vi "Send OOB TX.vi"(8 "error in (no error)":errorcluster, 11 "CIFCorePlugin in":refnum<class "CIFCorePlugin.lvclass">) -> (0 "error out":errorcluster, 3 "CIFCorePlugin out":refnum<class "CIFCorePlugin.lvclass">)   [LabVIEW 2021, in "CIFCorePlugin.lvclass"]
uses:
  CIFCorePlugin.lvclass
  CIFCorePlugin.lvclass/CIFCorePlugin.ctl
  CIFUtilities/CIFChannelMng/CIFChannelMng.lvclass/CIFChannelMng.ctl
  Common/Typedef/Plugin Overrides.ctl
  Common/Typedef/Timing Overrides.ctl
  Common/Typedef/Plugin Status.ctl
  Common/Typedef/Plugin State.ctl
  Common/Typedef/Timing Statistics.ctl
  Common/Typedef/Timing Stats Base.ctl
  Common/Typedef/FIFO Statistics.ctl
  Common/Typedef/Simple Error.ctl
  Common/Typedef/Monitor Doubles.ctl
  Common/Typedef/Monitor U64.ctl
  Common/Typedef/Monitor I64.ctl
  CIFUtilities/CIFOutOfBand/CIFOutOfBand.lvclass/CIFOutOfBand.ctl
  CIFUtilities/CIFOutOfBand/Write OOB DVR.vi
  CIFUtilities/CIFOutOfBand/Utilities/Command to Bitwise Command.vi
  CIFUtilities/CIFOutOfBand/Accessors/Read Local OOB Data.vi
  CIFUtilities/CIFOutOfBand/Accessors/Write Local OOB Data.vi
  CIFUtilities/CIFChannelMng/Accessors/Read Update OOB.vi
  CIFUtilities/CIFChannelMng/Accessors/Read Channel Status for OOB.vi
  CIFUtilities/CIFChannelMng/Accessors/Write Update OOB.vi
  OOB/OOB_Tx/CIFCoreOOB_Tx.lvclass
  D:/dev/CIF-LVCore/src/CIFUtilities/CIFOutOfBand/CIFOutOfBand.lvclass
  Common/CIFCoreCommon.lvlib
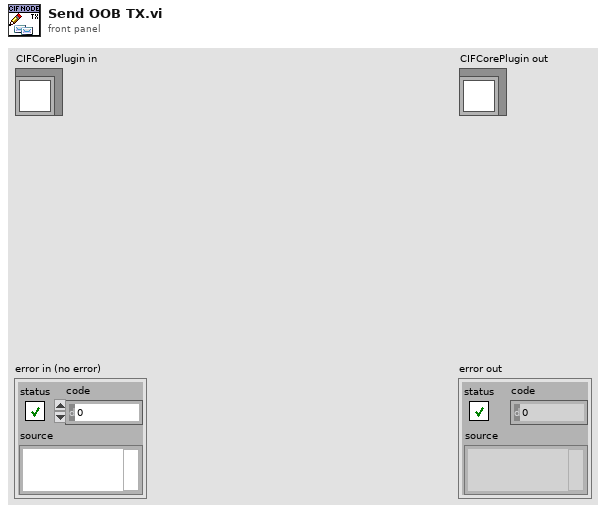
[diagram p1: front panel]
types:
  T1 = typedef "CIFCoreCommon.lvlib/Plugin Overrides.ctl" = cluster{"Timing Overrides":T2}
  T2 = typedef "CIFCoreCommon.lvlib/Timing Overrides.ctl" = cluster{"Override Timing":bool, "Skip Sleep":bool, "Period (s)":dbl}
  T3 = typedef "CIFCoreCommon.lvlib/Plugin Status.ctl" = cluster{"State":T4, "Timing Statistics (us)":T5, "FIFO Statistics (us)":T7, "error":T8, "Monitor Doubles":T9, "Monitor U64":T10, "Monitor I64":T11, "Cleanup":T6, "Create":i32, "Destroy":i32}
  T4 = typedef "CIFCoreCommon.lvlib/Plugin State.ctl" = enum32{"Null", "Creating", "Listening", "Running", "CleaningUp", "Destroying"}
  T5 = typedef "CIFCoreCommon.lvlib/Timing Statistics.ctl" = cluster{"Period":T6, "Wake Error":T6, "Execute":T6, "Housekeep":T6, "Idle":T6}
  T6 = typedef "CIFCoreCommon.lvlib/Timing Stats Base.ctl" = cluster{"Max":i32, "Min":i32}
  T7 = typedef "CIFCoreCommon.lvlib/FIFO Statistics.ctl" = cluster{"From T0":T6, "From Previous Plugin":T6, "Output Error":T6}
  T8 = typedef "CIFCoreCommon.lvlib/Simple Error.ctl" = cluster{"status":bool, "code":i32}
  T9 = typedef "CIFCoreCommon.lvlib/Monitor Doubles.ctl" = cluster{"1":dbl, "2":dbl, "3":dbl, "4":dbl}
  T10 = typedef "CIFCoreCommon.lvlib/Monitor U64.ctl" = cluster{"1":u64, "2":u64, "3":u64, "4":u64}
  T11 = typedef "CIFCoreCommon.lvlib/Monitor I64.ctl" = cluster{"1":i64, "2":i64, "3":i64, "4":i64}
  T12 = typedef "CIFChannelMng.lvclass/Channel List for OOB.ctl" = cluster{"Name":string, "Direction":T13, "Type":string, "Connected?":bool, "Connected Name":string, "Custom Config Data":u8[]}
  T13 = typedef "CIFChannels.lvclass/Direction.ctl" = enum16{"Publisher", "Subscriber"}
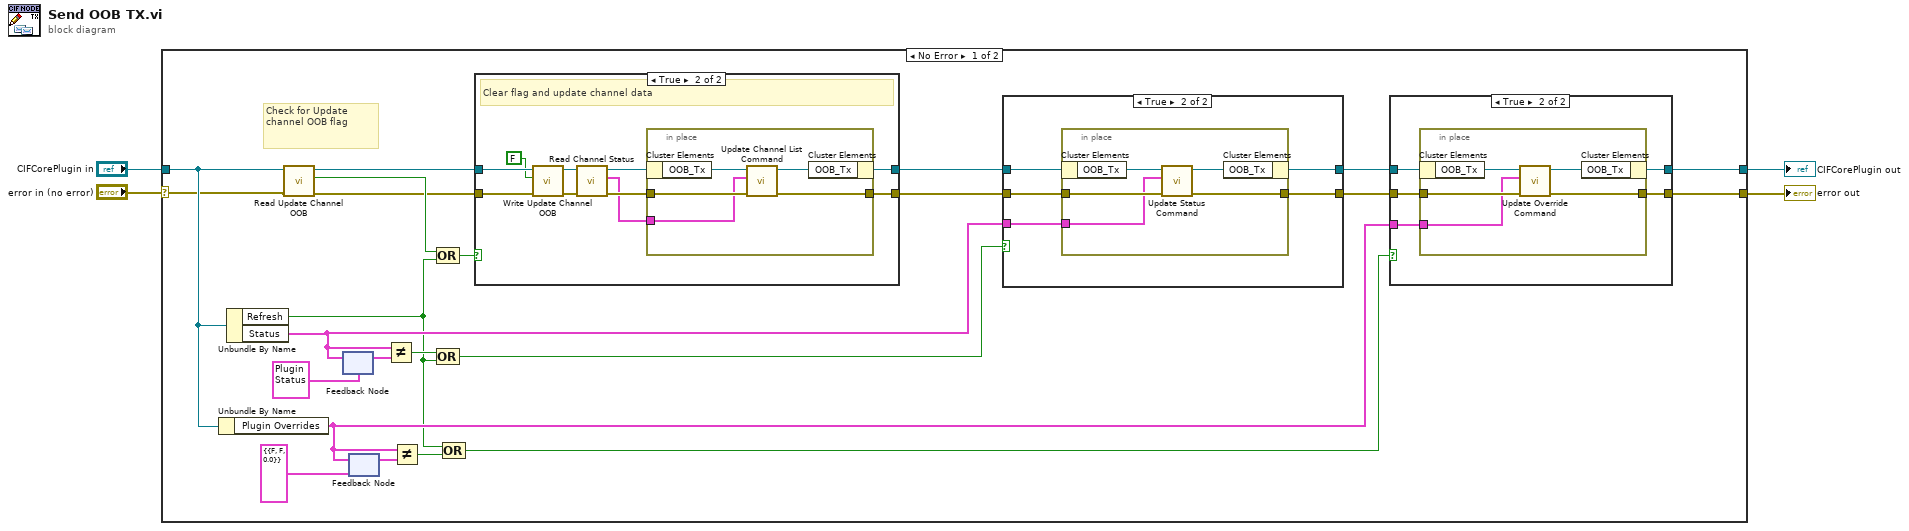
[diagram p0: block diagram]
diagram:
  n1 = case shown="No Error" "error in (no error)" {
    selector: "error in (no error)" -> [w10 w70]
    tunnel: [w6 w70] -> w3
    tunnel: [w7 w69] -> w1
    tunnel: "CIFCorePlugin in" -> [w13 w69]
    frame No Error {
      # "Check for Update channel OOB flag"
      n2 = Unbundle By Name(w13) -> ("Plugin Overrides"=w16:T1)
      n3 = Unbundle By Name(w13) -> ("Refresh"=w5:bool, "Status"=w24:T3)
      n4 = call "Read Update Channel OOB.vi"("error in (no error)"=w10, "CIFCorePlugin in"=w13) -> ("error out"=w9:errorcluster, "Update OOB"=w15:bool, "CIFCorePlugin out"=w11:refnum<class "CIFCorePlugin.lvclass">)  [unwired: 7 in]
      n5 = feedback-in #1(w24) -> ()
      n6 = feedback #1(T3 {"State"=enum."Null", "Timing Statistics (us)"={"Period"={"Max"=0, "Min"=0}, "Wake Error"={"Max"=0, "Min"=0}, "Execute"={"Max"=0, "Min"=0}, "Housekeep"={"Max"=0, "Min"=0}, "Idle"={"Max"=0, "Min"=0}}, "FIFO Statistics (us)"={"From T0"={"Max"=0, "Min"=0}, "From Previous Plugin"={"Max"=0, "Min"=0}, "Output Error"={"Max"=0, "Min"=0}}, "error"={"status"=FALSE, "code"=0}, "Monitor Doubles"={"1"=0.0, "2"=0.0, "3"=0.0, "4"=0.0}, "Monitor U64"={"1"=0, "2"=0, "3"=0, "4"=0}, "Monitor I64"={"1"=0, "2"=0, "3"=0, "4"=0}, "Cleanup"={"Max"=0, "Min"=0}, "Create"=0, "Destroy"=0} ("Status")) -> (w26:T3)
      n7 = feedback #2(T1 {"Timing Overrides"={"Override Timing"=FALSE, "Skip Sleep"=FALSE, "Period (s)"=0.0}} ("Plugin Overrides")) -> (w19:T1)
      n8 = feedback-in #2(w16) -> ()
      n9 = Not Equal?(x=w24, y=w26) -> (x != y?=w25:bool)
      n10 = Not Equal?(x=w16, y=w19) -> (x != y?=w20:bool)
      n11 = Compound Arithmetic op=OR(w15, w5) -> (w8:bool)
      n12 = Compound Arithmetic op=OR(w25, w5) -> (w23:bool)
      n13 = Compound Arithmetic op=OR(w5, w20) -> (w17:bool)
      n14 = case shown="True" w8 {
        tunnel: w9 -> [w28 w33]
        tunnel: w11 -> [w29 w34]
        tunnel: [w29 w39] -> w14
        tunnel: [w28 w38] -> w12
        frame False {
        }
        frame True {
          # "Clear flag and update channel data"
          n15 = call "Write Update Channel OOB.vi"("error in (no error)"=w33, "Update OOB"=FALSE, "CIFCorePlugin in"=w34) -> ("error out"=w31:errorcluster, "CIFCorePlugin out"=w32:refnum<class "CIFCorePlugin.lvclass">)  [unwired: 7 in]
          n16 = call "Read Channel Status.vi"("error in (no error)"=w31, "CIFCorePlugin in"=w32) -> ("error out"=w36:errorcluster, "Channel Status"=w35:T12[], "CIFCorePlugin out"=w37:refnum<class "CIFCorePlugin.lvclass">)  [unwired: 7 in]
          n17 = in-place {
            in-place-border: w36 -> [w42]
            in-place-border: [w41] -> w38
            in-place-border: w35 -> [w40]
            n18 = in-place-cluster #3(w37) -> ("OOB_Tx"=w44:refnum<class "CIFCoreOOB_Tx.lvclass">)
            n19 = call "Update Channel List Command.vi"("error in"=w42, "Channel List"=w40, "CoreOOB_Tx in"=w44) -> ("error out"=w41:errorcluster, "CoreOOB_Tx out"=w43:refnum<class "CIFCoreOOB_Tx.lvclass">)  [unwired: 7 in]
            n20 = in-place-cluster #3("OOB_Tx"=w43) -> (w39:refnum<class "CIFCorePlugin.lvclass">)
          }
        }
      }
      n21 = case shown="True" w23 {
        tunnel: w12 -> [w57 w63]
        tunnel: w14 -> [w58 w62]
        tunnel: w24 -> [_ w61]
        tunnel: [w58 w60] -> w22
        tunnel: [w57 w59] -> w21
        frame False {
        }
        frame True {
          n22 = in-place {
            in-place-border: w63 -> [w66]
            in-place-border: [w65] -> w59
            in-place-border: w61 -> [w64]
            n23 = in-place-cluster #4(w62) -> ("OOB_Tx"=w68:refnum<class "CIFCoreOOB_Tx.lvclass">)
            n24 = call "Update Status Command.vi"("error in"=w66, "Status"=w64, "CoreOOB_Tx in"=w68) -> ("error out"=w65:errorcluster, "CoreOOB_Tx out"=w67:refnum<class "CIFCoreOOB_Tx.lvclass">)  [unwired: 7 in]
            n25 = in-place-cluster #4("OOB_Tx"=w67) -> (w60:refnum<class "CIFCorePlugin.lvclass">)
          }
        }
      }
      n26 = case shown="True" w17 {
        tunnel: w21 -> [w45 w51]
        tunnel: w22 -> [w46 w50]
        tunnel: w16 -> [_ w49]
        tunnel: [w46 w48] -> w7
        tunnel: [w45 w47] -> w6
        frame False {
        }
        frame True {
          n27 = in-place {
            in-place-border: w51 -> [w54]
            in-place-border: [w53] -> w47
            in-place-border: w49 -> [w52]
            n28 = in-place-cluster #5(w50) -> ("OOB_Tx"=w56:refnum<class "CIFCoreOOB_Tx.lvclass">)
            n29 = call "Update Override Command.vi"("error in"=w54, "Plugin Overrides"=w52, "CoreOOB_Tx in"=w56) -> ("error out"=w53:errorcluster, "CoreOOB_Tx out"=w55:refnum<class "CIFCoreOOB_Tx.lvclass">)  [unwired: 7 in]
            n30 = in-place-cluster #5("OOB_Tx"=w55) -> (w48:refnum<class "CIFCorePlugin.lvclass">)
          }
        }
      }
    }
    frame Error {
    }
  }
  "error out" <- w3
  "CIFCorePlugin out" <- w1
